vi "Limits from tolerance.vi"(9 "Nominal":dbl, 10 "Tolerance %":dbl) -> (1 "Min Limit":dbl, 2 "Max Limit":dbl)   [LabVIEW 2018]
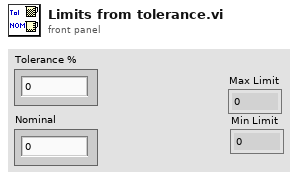
[diagram p1: front panel]
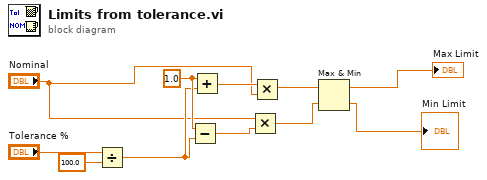
[diagram p0: block diagram]
diagram:
  w9 = 1.0 ("x")
  n1 = Divide(x="Tolerance %", y=100.0) -> (x/y=w8:dbl)
  n2 = Subtract(x=w9, y=w8) -> (x-y=w7:dbl)
  n3 = Add(x=w9, y=w8) -> (x+y=w6:dbl)
  n4 = Multiply(x="Nominal", y=w7) -> (x*y=w3:dbl)
  n5 = Multiply(x=w6, y="Nominal") -> (x*y=w4:dbl)
  n6 = Max & Min(x=w4, y=w3) -> (max(x,y)=→"Max Limit":dbl, min(x,y)=→"Min Limit":dbl)
